vi "Actor Core.vi"(8 "error in":errorcluster, 11 "UART Actor in":refnum<class "UART Actor.lvclass">) -> (0 "error out":errorcluster, 3 "Actor out":refnum<class "Actor.lvclass">)   [LabVIEW 2020, in "UART Actor.lvlib" / "UART Actor.lvclass"]
doc: "(<B>Filename</B>: Actor Framework.lvlib:Actor.lvclass:Actor Core.vi)\n\nReceives messages to the actor, reacts to them, and initiates any error handling that may shut the actor down.\n\nDescendant classes may override this VI to append parallel tasks for the actor to complete while it handles messages. Overrides use the Call Parent Class Method node."
uses:
  UART Actor.lvclass
  C:/Program Files (x86)/National Instruments/LabVIEW 2020/vi.lib/ActorFramework/Actor/Actor.lvclass
  <vilib>/ActorFramework/Actor/Actor.lvclass
  <vilib>/ActorFramework/Actor/Actor.lvclass/Actor.ctl
  <vilib>/ActorFramework/Message Enqueuer/Message Enqueuer.lvclass/Message Enqueuer.ctl
  UART Actor Messages/Open Port Msg/Open Port Msg.lvclass/Open Port Msg.ctl
  UART Actor Messages/Write Buffer Msg/Write Buffer Msg.lvclass/Write Buffer Msg.ctl
  <vilib>/ActorFramework/Message Enqueuer/Init from Existing Queue.vi
  <vilib>/ActorFramework/Message Enqueuer/Enqueue.vi
  <vilib>/ActorFramework/Stop Msg/Stop Msg.lvclass
  C:/Program Files (x86)/National Instruments/LabVIEW 2020/vi.lib/ActorFramework/Message/Message.lvclass
  UART Actor Messages/Close Port Msg/Close Port Msg.lvclass
  UART Actor Messages/Open Port Msg/Open Port Msg.lvclass
  UART Actor Messages/Write Buffer Msg/Write Buffer Msg.lvclass
  <vilib>/ActorFramework/Message Priority Queue/Priority Enqueue.vi
  <vilib>/ActorFramework/Message Enqueuer/Message Enqueuer.lvclass
  UART Actor.lvclass/UART Actor.ctl
panel:
  in  "stop":bool
  in  "讀取目標字數":i32=1
  in  "Write":bool
  in  "VISA resource name":refnum<visa-resource-name>
  out "read buffer":string
  in  "write buffer":string
  # "1. 設定 VISA\n2. 設定讀取目標字數\n3. 按下”開始通訊”，進行通訊作業\n4. 設定\"write buffer“\n5. 按下\"Write\"，將資料進行寫入\n6. 觀察\"read buffer\"\n7. 按下停止通訊“，結束通訊作業"
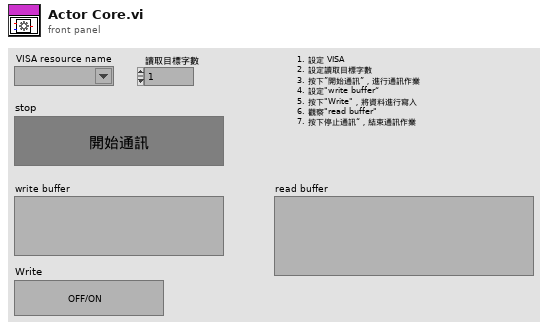
[diagram p1: front panel]
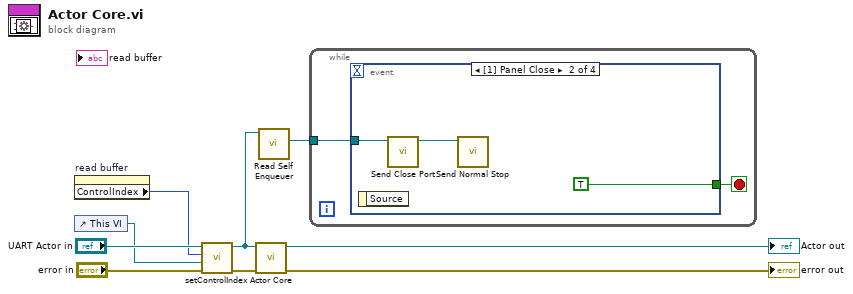
[diagram p0: block diagram]
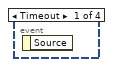
[diagram p2: hidden frame]
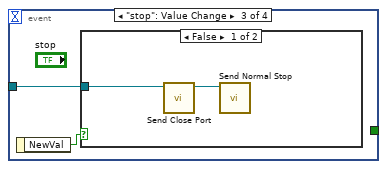
[diagram p3: hidden frame]
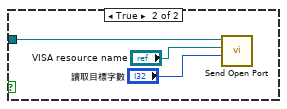
[diagram p4: hidden frame]
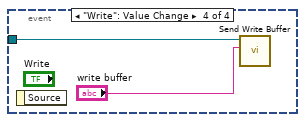
[diagram p5: hidden frame]
diagram:
  n1 = property on="read buffer" class="Str"() -> ("ControlIndex"=w2:i32)  [unwired: 2 in, 2 out]
  n2 = control-ref of="This VI"() -> (w1:refnum<vi>)
  n3 = call "setControlIndex.vi"("error in (no error)"="error in", "VI Refnum"=w1, "readBufferControlIndex"=w2, "UART Actor in"="UART Actor in") -> ("error out"=w3:errorcluster, "UART Actor out"=w5:refnum<class "UART Actor.lvclass">)  [unwired: 6 in]
  n4 = call-parent "Actor Core.vi"("error in"=w3, "Actor in"=w5) -> ("error out"=→"error out":errorcluster, "Actor out"=→"Actor out":refnum<class "Actor.lvclass">)  [unwired: 8 in]
  n5 = call <vilib>:"Read Self Enqueuer.vi"("Actor"=w5) -> ("Self Enqueuer"=w7:refnum<class "Message Enqueuer.lvclass">)  [unwired: 10 in]
  n6 = while {
    tunnel: w7 -> [w10]
    stop <- w11 stop-if-true
    n7 = event shown="[1] Panel Close" {
      selector: _ -> [_ _ _ _]
      dyn-events: _ -> [_ _ _ _]
      timeout: _ -> [_ _ _ _]
      tunnel: [_ TRUE _ _] -> w11
      tunnel: w10 -> [_ w13 w16 w23]
      event Timeout {
        n8 = event-data() -> ()  [unwired: 1 in, 1 out]
      }
      event Panel Close {
        n9 = event-data() -> ()  [unwired: 1 in, 1 out]
        n10 = call "Send Close Port.vi"("Message Enqueuer"=w13) -> ("Message Enqueuer out"=w12:refnum<class "Message Enqueuer.lvclass">)  [unwired: 9 in, 1 out]
        n11 = call <vilib>:"Send Normal Stop.vi"("Message Enqueuer"=w12) -> ()  [unwired: 10 in, 1 out]
      }
      event "stop": Value Change {
        n12 = event-data() -> ("NewVal"=w15:bool)  [unwired: 1 in]
        n13 = case shown="False" w15 {
          tunnel: w16 -> [w18 w21]
          frame False {
            n14 = call "Send Close Port.vi"("Message Enqueuer"=w18) -> ("Message Enqueuer out"=w17:refnum<class "Message Enqueuer.lvclass">)  [unwired: 9 in, 1 out]
            n15 = call <vilib>:"Send Normal Stop.vi"("Message Enqueuer"=w17) -> ()  [unwired: 10 in, 1 out]
          }
          frame True {
            n16 = call "Send Open Port.vi"("targetCount"="讀取目標字數", "VISA"="VISA resource name", "Message Enqueuer"=w21) -> ()  [unwired: 7 in, 2 out]
          }
        }
      }
      event "Write": Value Change {
        n17 = event-data() -> ()  [unwired: 1 in, 1 out]
        n18 = call "Send Write Buffer.vi"("write buffer"="write buffer", "Message Enqueuer"=w23) -> ()  [unwired: 8 in, 2 out]
      }
    }
  }
